vi "Set-available-actions.vi"(8 "error in (no error)":errorcluster, 10 "Supported actions":T2[](array[typedef]), 11 "Data in":T1) -> (0 "error out":errorcluster, 3 "Data out":T1)   [LabVIEW 2013, in "PowderDeposition.lvlib" / "PD-Main.lvclass"]
doc: "Takes the list of a motor's supported actions and disables only the non-supported\nactions in the GUI's action selector. Sets the action selector value to the first action in\n the supported actions list."
uses:
  PD-Main.lvclass
  Object-reference.ctl
  Action/Motor-actions.ctl
  PD-Main.lvclass/PD-Main.ctl
  Read Actions.vi
  Action/Action.lvclass
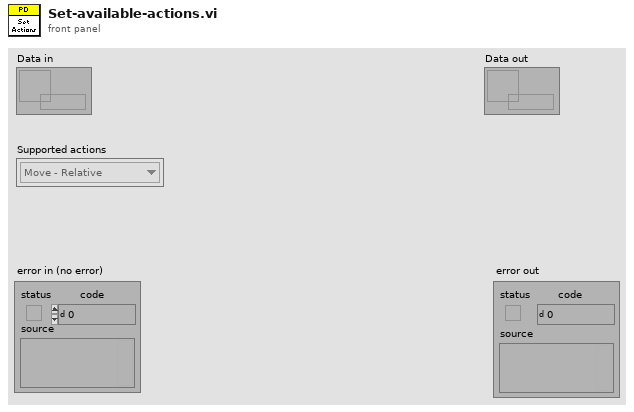
[diagram p1: front panel]
types:
  T1 = typedef "PowderDeposition.lvlib/PD-Main.lvclass/Object-reference.ctl" = refnum<data-value>
  T2 = typedef "PowderDeposition.lvlib/Action.lvclass/Motor-actions.ctl" = enum16{"Move - Absolute", "Move - Relative", "Move - Timer", "Wait", "Home", "Substrate", "Sieve", "Stop"}
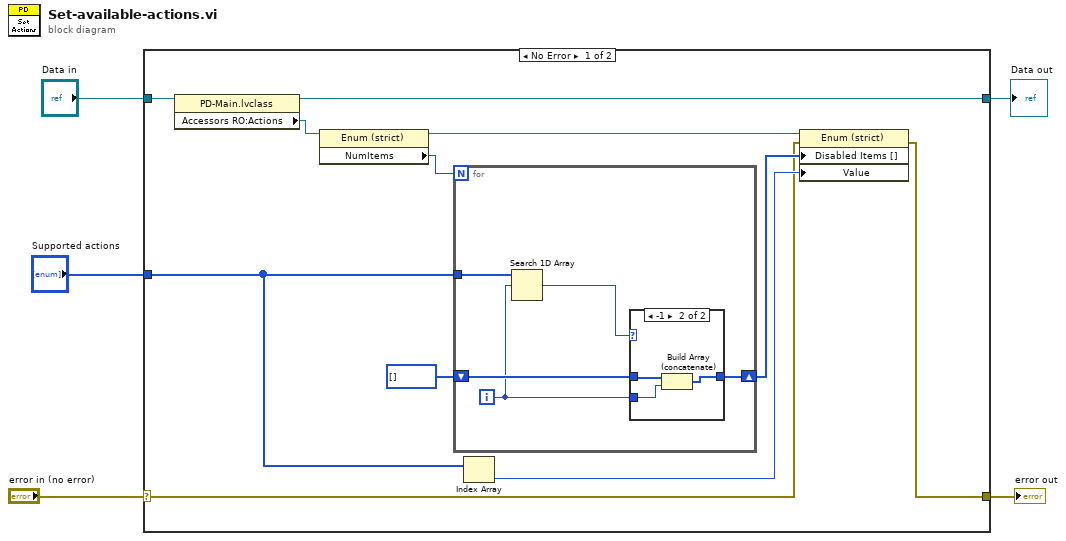
[diagram p0: block diagram]
diagram:
  n1 = case shown="No Error" "error in (no error)" {
    selector: "error in (no error)" -> [w8 w27]
    tunnel: [w7 w27] -> w4
    tunnel: "Data in" -> [w14 w26]
    tunnel: "Supported actions" -> [w10 _]
    tunnel: [w12 w26] -> w1
    frame No Error {
      n2 = property class="PD-Main.lvclass"(reference=w14) -> (reference out=w12:T1, "Accessors RO:Actions"=w11:refnum<vi>)  [unwired: 1 in, 1 out]
      n3 = property class="Enum (strict)"(reference=w11) -> (reference out=w6:refnum<vi>, "NumItems"=w9:u32)  [unwired: 1 in, 1 out]
      n4 = for {
        N: w9 -> [_]
        shift-right: [w20] -> w15
        shift-left: i32[] [] -> [w21]
        tunnel: w10 -> [w19]
        i -> [w18]
        n5 = Search 1D Array(1D array=w19, element=w18) -> (index of element=w17:i32)  [unwired: 1 in]
        n6 = case shown="-1" w17 {
          tunnel: w18 -> [_ w23]
          tunnel: w21 -> [w22 w25]
          tunnel: [w22 w24] -> w20
          frame Default {
          }
          frame -1 {
            n7 = Build Array (concatenate)(w25, w23) -> (w24:i32[])
          }
        }
      }
      n8 = Index Array(array=w10) -> (element=w13:T2)  [unwired: 1 in]
      n9 = property class="Enum (strict)"(reference=w6, error in=w8, "Disabled Items []"=w15, "Value"=w13) -> (error out=w7:errorcluster)  [unwired: 1 out]
    }
    frame Error {
    }
  }
  "error out" <- w4
  "Data out" <- w1
